vi "TESTE.vi"() -> ()   [LabVIEW 2018]
uses:
  CCDCamera/CCDCamera.lvclass
  <userlib>/atmcd32d.llb/Shutter_mode typedef.ctl
  <userlib>/atmcd32d.llb/HSSpeed_type typedef.ctl
  <userlib>/atmcd32d.llb/AcquisitionMode_mode typedef.ctl
  <userlib>/atmcd32d.llb/TriggerMode_mode typedef.ctl
  <userlib>/atmcd32d.llb/ReadMode_mode typedef.ctl
  <userlib>/atmcd32d.llb/Shutter_type typedef.ctl
  <userlib>/gfitsio/gfitsio.lvlib
  <userlib>/gfitsio/cfitsio-bitpix.ctl
  <userlib>/gfitsio/gfitsio-write-key-string.vi
  <userlib>/gfitsio/gfitsio-write-image-subset-variant.vi
  Save Image/Save Image.lvclass
  Sync Box/Sync Box.lvclass
panel:
  out "data out":string
  in  "Array 2":u16[](array[numeric])
  in  "CCD Config":T1={"Exposure Time"=0.1, "Pre-amp gain"=0, "Readout Rate"=0, "EM Mode"=0, "EM Gain"=2, "Binning"=1, "Initial Line"=1, "Initial Cloumn"=1, "Final Line"=1024, "Final Column"=1024, "Kinetic Series Length"=1, "Shutter Mode"=0, "Cooler ON/OFF"=0, "Temperature"=20, "Image Name"="", "Image Path"="", "Current Temperature"=0, "Temperatue Status"="", "Serial Number"=0, "#image"=1} {"Pre-amp gain" items=["Gain 1", "Gain 2"]; "Readout Rate" items=["1 MHz", "10 MHz", "20 MHz", "30 MHz"]; "EM Mode" items=["Electron Multiplying", "Conventional"]}
  in  "Array":u16[][][](array[numeric])=[[[1, 2], [3, 4]], [[5, 6], [7, 8]], [[4, 7], [8, 7]]]
  out "array":u16[][][](array[numeric])
  out "last":u8
  out "first":u8
  in  "CCDCamera.lvclass":refnum<class "CCDCamera.lvclass">
  out "speed":sgl format="%.2f"
  in  "Header Contents":T2={"FILENAME"=["FILENAME", "Image", "File name at acquisition"], "OBSERVER"=["OBSERVER", "Anonymous", "Name of the observer"], "PROGRID"=["PROGRID", "2018A-001", "Program ID"], "OBJECT"=["OBJECT", "UNDEFINED", "Object name"], "NIGHTDIR"=["NIGHTDIR", "C:\\Users\\observer\\Desktop\\SPARC4 Acquisition Control\\Imagens\\", "Night directory name "], "CHANNEL"=["CHANNEL", "1", "Instrument channel"], "INSTRUME"=["INSTRUME", "SPARC4", "Instrument"], "NEXPSEQ"=["NEXPSEQ", "1", "Total number of exposures in sequence"], "SEQINDEX"=["SEQINDEX", "1", "Exposure index in the sequence"], "OBSTYPE"=["OBSTYPE", "BIAS", "Image type: OBJECT, BIAS, FLAT, ARC, DARK"], "READMOD"=["READMOD", "Normal", "Read out mode: fast, normal, slow"], "READMODE"=["READMODE", "Image", "CCD read mode"], "ACQMODE"=["ACQMODE", "Kinetic", "Acquisition Mode"], "PREAMP"=["PREAMP", "Gain 1", "Pre-amplifier gain"], "READOUT"=["READOUT", "30 MHz", "Readout Rate"], "VSHIFT"=["VSHIFT", "4.33", "Vertical Shift Speed"], "TRIGGER"=["TRIGGER", "Internal", "Trigger Mode"], "EMMODE"=["EMMODE", "Electron Multiplying", "Output amplifier mode"], "EMGAIN"=["EMGAIN", "2", "EM Gain"], "VBIN"=["VBIN", "1", "Vertical binning"], "HBIN"=["HBIN", "1", "Horizontal binning"], "INITLINE"=["INITLIN", "1", "Initial Line"], "INITCOL"=["INITCOL", "1", "Initial Column"], "FINALLIN"=["FINALIN", "1024", "Final Line"], "FINALCOL"=["FINALCOL", "1", "Final Column"], "KSERLEN"=["KSERLEN", "CLOSED", "Kinetic Series Length"], "SHUTTER"=["SHUTTER", "50", "Shutter Mode (OPEN, CLOSED, or AUTO) "], "OPENSHT"=["OPENSHT", "50", "Time to open the shutter (ms) "], "CLOSESHT"=["CLOSESHT", "2019-03-14T14:55:35.63", "Time to close the shutter (ms)"], "DATE"=["DATE", "3.38", "Date of the acquired image (YY/MM/DD:HH:MM:SS.sss"], "GAIN"=["GAIN", "0.05", "Gain (e-/ADU)"], "GAINERR "=["GAINERR", "6.55", " Gain error (e-/ADU)"], "RDNOISE"=["RDNOISE", "0.02", "Read noise (e-)"], "RNOISERR"=["RNOISERR", "OFF", "Read noise error (e-)"], "SKYFIBER"=["SKYFIBER", "OFF", "Sky fiber: ON or OFF"], "CALFIBER"=["CALFIBER", "2017-10-01T20", "Calibration Fiber: ON or OFF"], "UTDATE"=["UTDATE", "2017-10-01T17", "UT date at start of exposure"], "LOCTIME"=["LOCTIME", "58027.500000", "LT date at start of exposure"], "MJD"=["MJD", "-45.57972", "Modified Julian Date at start of exposure"], "OBSLON"=["OBSLON", "-22.53444", "Observatory East Longitude"], "OBSLAT"=["OBSLAT", "1864.0", "Observatory Latitude"], "OBSALT"=["OBSALT", "0", "Observatory elevation above sea level (m)"], "EXPTIME"=["EXPTIME", "0000:00.000", "Exposure time (s)"], "TELRA"=["TELRA", "+00:00:00.000", "TCS right ascension: HH:MM:SS.SSS"], "TELDEC"=["TELDEC", "00:00:00.000", "TCS declination: +-DD:MM:SS.SSS"], "RA"=["RA", "+00:00:00.000", "Requested right Ascension: HH:MM:SS.SSS"], "DEC"=["DEC", "128.84946", "Requested Declination: +- DD:MM:SS.SSS"], "RA_DEG"=["RA_DEG", "+19.648717", "Requested Right Ascension (deg)"], "DEC_DEG"=["DEC_DEG", "2000.00", "Requested Declination (deg)"], "EPOCH"=["EPOCH", "+01:13:05.98", "Epoch for Target coordinates"], "HA"=["HA", "1.2183292", "Hour Angle (Sexagesimal)"], "HAD"=["HAD", "1.085", "Hour Angle (deg)"], "AIRMASS"=["AIRMASS", "1.060", "Mean airmass for the observation"], "AMSTART"=["AMSTART", "1.114", "Airmass at start of exposure"], "AMEND"=["AMEND", "0.000000", "Airmass at end of exposure"], "XOFFSET"=["XOFFSET", "0.000000", "Telescope RA offset in arcsec"], "YOFFSET"=["YOFFSET", "14.6415392418", "Telescope DEC offset in arcsec"], "PA"=["PA", "-3.53", "Current Rotator Position Angle (degree)"], "CAMFOC"=["CAMFOC", "-3.53", "Camera focus position (mm)"], "TELFOC"=["TELFOC", "23:17:24.8", "Telescope focus position (mm)"], "TCSUT"=["TCSUT", "23:12:32.5", "TCS Universal Time"], "TCSST"=["TCSST", "15.0", "TCS Sideral Time"], "MOONDIST"=["MOONDIST", "60.0", "Moon angular distance to object (deg)"], "MOONALT"=["MOONALT", "15.0", "Moon elevation above horizon (deg)"], "MOONPHAS"=["MOONPHAS", "30.0", "Moon phase (deg)"], "ADC"=["ADC", "OFF", "Atmospheric Dispersion Corrector: ON or OFF"], "ADCSPEED"=["ADCSPEED", "0", "ADC motor speed (rpm)"], "CALMIRR"=["CALMIRR", "OUT", "Calibration mirror position: IN or OUT"], "GUIDING"=["GUIDING", "OFF", "Guider status: ON or OFF"], "GUIDTEXP"=["GUIDTEXP", "0", "Guider exposure time (s)"], "GUIDFREQ"=["GUIDFREQ", "0", "Guiding frequency (Hz)"], "GUIDOBJX"=["GUIDOBJX", "102.5", "Guiding object x position (pixel)"], "GUIDOBJY"=["GUIDOBJY", "300.3", "Guiding object y position (pixel)"], "AVGYCORR"=["AVGYCORR", "2.3", "Average correction in RA (arcsec)"], "AVGXCORR"=["AVGXCORR", "1.3", "Average correction in DEC (arcsec)"], "GFOCUS"=["GFOCUS", "3.0", "Guider focus position (mm)"], "THARLAMP"=["THARLAMP", "OFF", "Thorium-Argon lamp state: ON or OFF"], "HALLAMP"=["HALLAMP", "OFF", "Halogen lamp state: ON or OFF"], "AGITATOR"=["AGITATOR", "OFF", "Fiber agitator: ON or OFF"], "THARMIRR"=["THARMIRR", "OFF", "Th-Ar mirror position: SPECTROGRAPH or TELESCOPE"], "DSTATUS"=["DSTATUS", "SPECTROGRAPH", "Dome Status: OPEN or CLOSED"], "DTEMP"=["DTEMP", "OPEN", "Dome temperature (deg C)"], "DHUM"=["DHUM", "0.00000", "Dome humidity (per cent)"], "DLAMP"=["DLAMP", "10.0", "Dome lamp: ON or OFF"], "DFLAT"=["DFLAT", "82.0", "Dome flat lamp: ON or OFF"], "TEMPEXT"=["TEMPEXT", "OFF", "External temperature (deg C)"], "PRESSURE"=["PRESSURE", "OFF", "Pressure (mbar)"], "HUMIDITY"=["HUMIDITY", "10.0", "Humidity (per cent)"], "WINDDIR"=["WINDDIR", "742.00", "Wind direction: North-eastward (deg)"], "WSPEED"=["WSPEED", "92.00", "Wind Speed (km/h)"], "DPOS"=["DPOS", "30.2", "Dome position (deg)"], "SHTTTL"=["SHTTTL", "TTL LOW", "Shutter TTL"]}
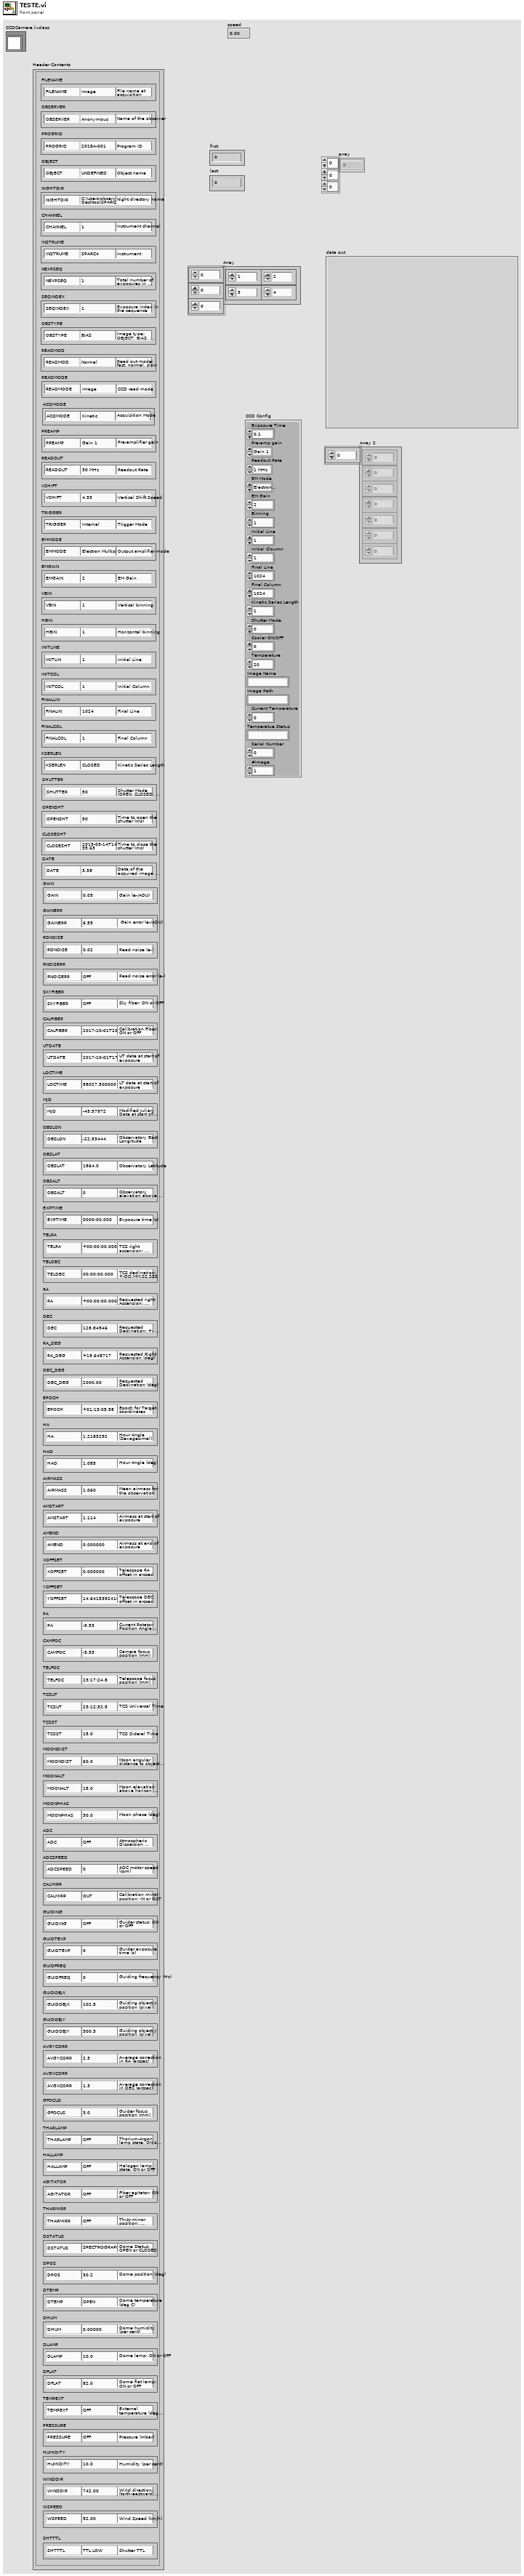
[diagram p1: front panel]
types:
  T1 = cluster{"Exposure Time":sgl, "Pre-amp gain":u8, "Readout Rate":u8, "EM Mode":u8, "EM Gain":u16, "Binning":u16, "Initial Line":u16, "Initial Cloumn":u16, "Final Line":u16, "Final Column":u16, "Kinetic Series Length":u32, "Shutter Mode":u8, "Cooler ON/OFF":u8, "Temperature":i8, "Image Name":string, "Image Path":string, "Current Temperature":i16, "Temperatue Status":string, "Serial Number":u16, "#image":u32}
  T2 = cluster{"FILENAME":string[], "OBSERVER":string[], "PROGRID":string[], "OBJECT":string[], "NIGHTDIR":string[], "CHANNEL":string[], "INSTRUME":string[], "NEXPSEQ":string[], "SEQINDEX":string[], "OBSTYPE":string[], "READMOD":string[], "READMODE":string[], "ACQMODE":string[], "PREAMP":string[], "READOUT":string[], "VSHIFT":string[], "TRIGGER":string[], "EMMODE":string[], "EMGAIN":string[], "VBIN":string[], "HBIN":string[], "INITLINE":string[], "INITCOL":string[], "FINALLIN":string[], "FINALCOL":string[], "KSERLEN":string[], "SHUTTER":string[], "OPENSHT":string[], "CLOSESHT":string[], "DATE":string[], "GAIN":string[], "GAINERR ":string[], "RDNOISE":string[], "RNOISERR":string[], "SKYFIBER":string[], "CALFIBER":string[], "UTDATE":string[], "LOCTIME":string[], "MJD":string[], "OBSLON":string[], "OBSLAT":string[], "OBSALT":string[], "EXPTIME":string[], "TELRA":string[], "TELDEC":string[], "RA":string[], "DEC":string[], "RA_DEG":string[], "DEC_DEG":string[], "EPOCH":string[], "HA":string[], "HAD":string[], "AIRMASS":string[], "AMSTART":string[], "AMEND":string[], "XOFFSET":string[], "YOFFSET":string[], "PA":string[], "CAMFOC":string[], "TELFOC":string[], "TCSUT":string[], "TCSST":string[], "MOONDIST":string[], "MOONALT":string[], "MOONPHAS":string[], "ADC":string[], "ADCSPEED":string[], "CALMIRR":string[], "GUIDING":string[], "GUIDTEXP":string[], "GUIDFREQ":string[], "GUIDOBJX":string[], "GUIDOBJY":string[], "AVGYCORR":string[], "AVGXCORR":string[], "GFOCUS":string[], "THARLAMP":string[], "HALLAMP":string[], "AGITATOR":string[], "THARMIRR":string[], "DSTATUS":string[], "DTEMP":string[], "DHUM":string[], "DLAMP":string[], "DFLAT":string[], "TEMPEXT":string[], "PRESSURE":string[], "HUMIDITY":string[], "WINDDIR":string[], "WSPEED":string[], "DPOS":string[], "SHTTTL":string[]}
  T3 = typedef "Shutter_mode typedef.ctl" = enum16{"Auto", "Open", "Close", "N/A (3)", "Open FVB Series", "Open Any Series"}
  T4 = typedef "AcquisitionMode_mode typedef.ctl" = enum16{"Reserved (0)", "Single Scan", "Accumulate", "Kinetics", "Fast Kinetics", "Run Till Abort", "Reserved (6)", "Reserved (7)", "Reserved (8)", "Time Delayed Integration"}
  T5 = typedef "TriggerMode_mode typedef.ctl" = enum16{"Internal", "External", "N/A (2)", "N/A (3)", "N/A (4)", "N/A (5)", "External Start", "External Exposure (Bulb)", "N/A (8)", "External FVB EM", "Software", "N/A (11)", "External Charge Shifting"}
  T6 = typedef "ReadMode_mode typedef.ctl" = enum16{"Full Vertical Binning", "Multi-Track", "Random-Track", "Single-Track", "Image"}
  T7 = typedef "Shutter_type typedef.ctl" = enum16{"TTL Low", "TTL High"}
  T8 = typedef "HSSpeed_type typedef.ctl" = enum16{"EM Amp", "Conventional Amp"}
  T9 = enum16{"open", "open or create", "create", "create or replace"}
  T10 = enum16{"open", "open or create", "create or replace", "create", "open (read only)"}
  T11 = typedef "gfitsio.lvlib/cfitsio-bitpix.ctl" = i32
  T12 = typedef "gfitsio.lvlib/gfitsio-refnum.ctl" = refnum<k1>
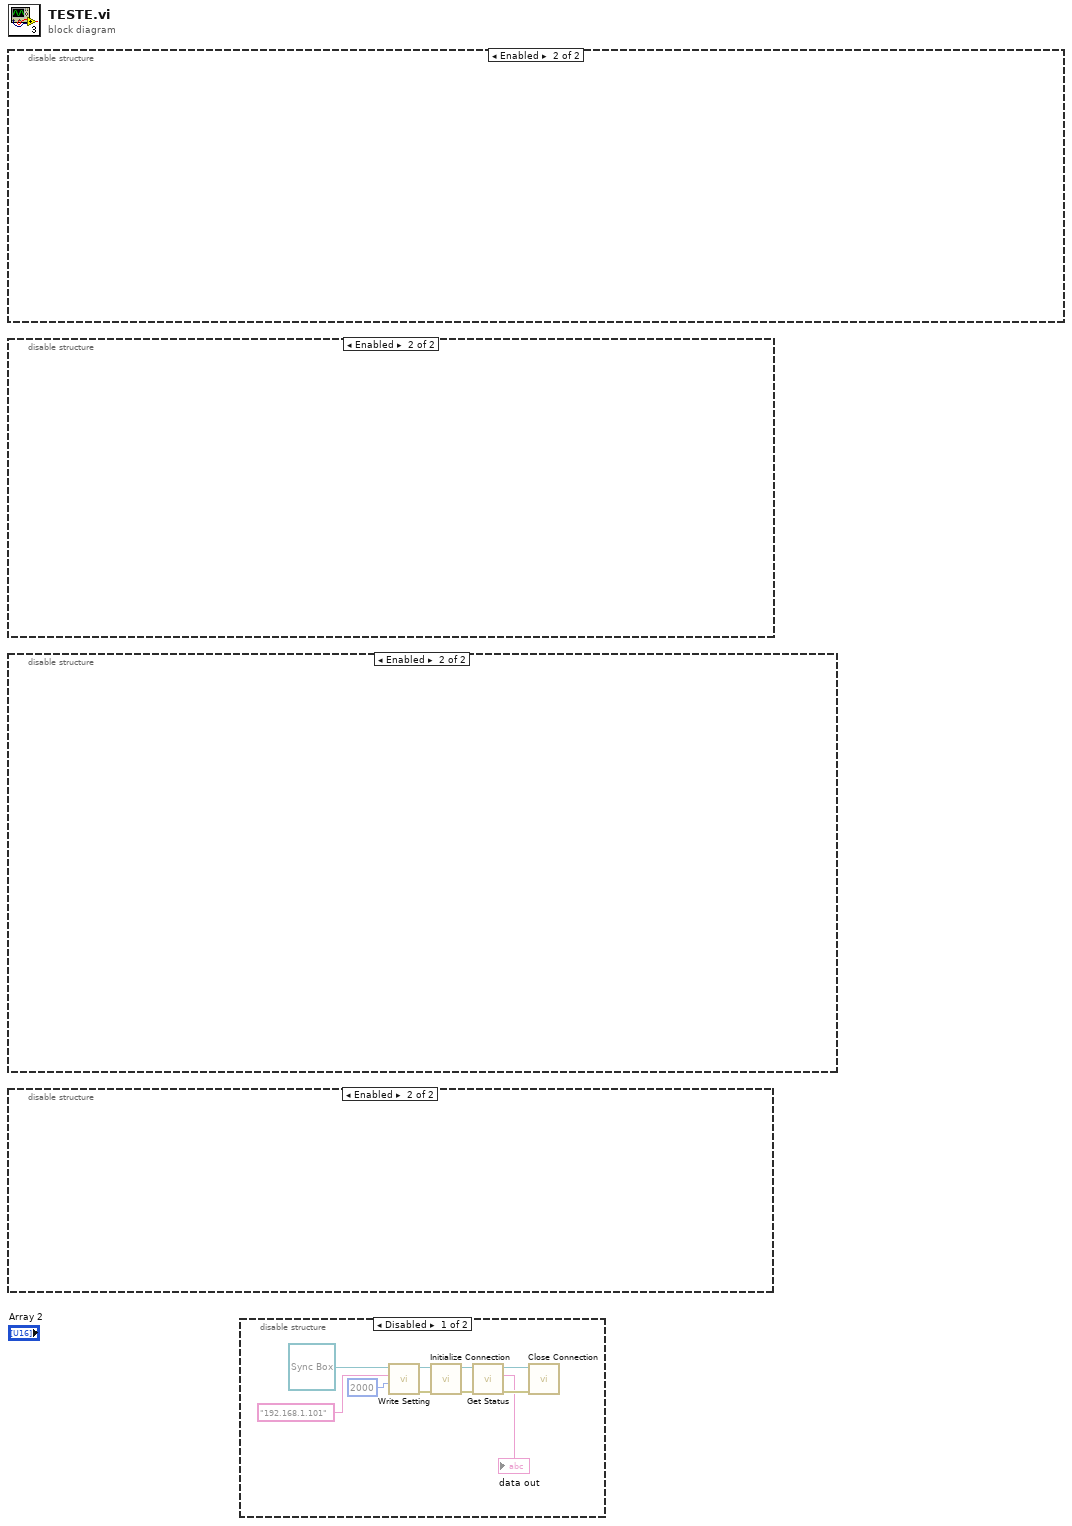
[diagram p0: block diagram]
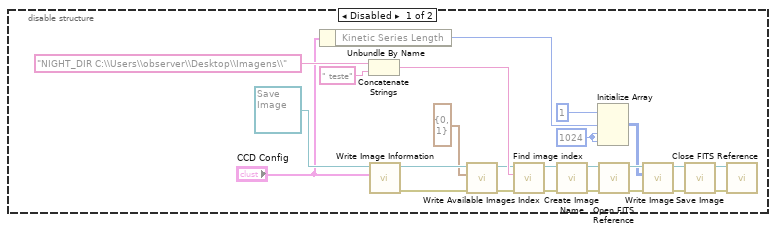
[diagram p3: hidden frame]
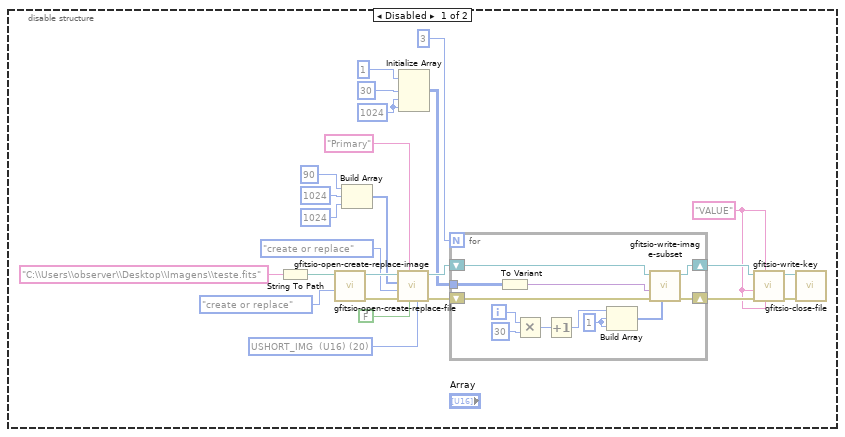
[diagram p4: hidden frame]
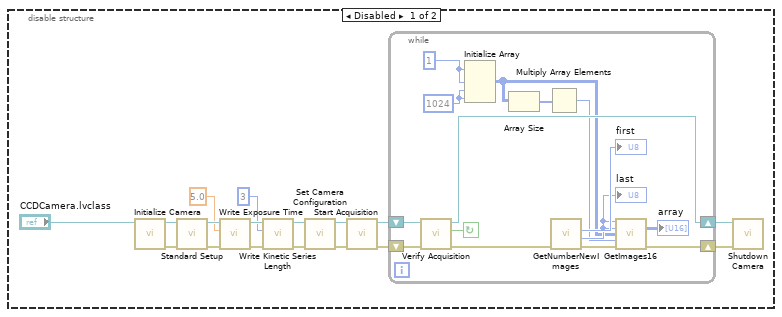
[diagram p5: hidden frame]
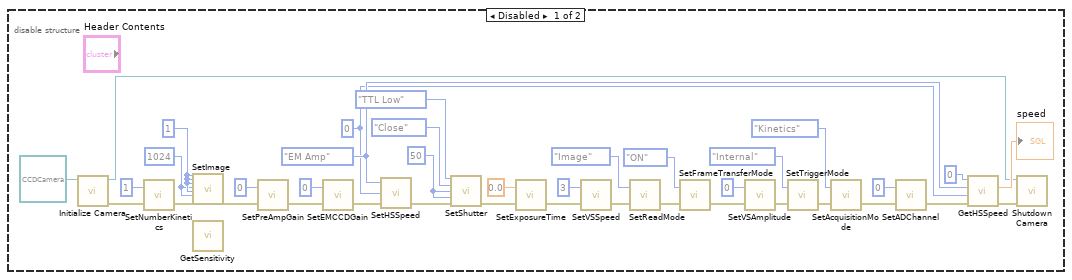
[diagram p6: hidden frame]
diagram:
  n1 = disable-structure shown="Enabled" {
    frame Disabled {
      w2 = HSSpeed_type_typedef."EM Amp" ("type")
      w1 = 0 ("index")
      w12 = 1024 ("number")
      w13 = 1 ("number")
      w28 = 50 ("openingtime")
      n2 = call "Initialize Camera.vi"("CCDCamera in"=refnum<class "CCDCamera.lvclass"> refnum ("CCDCamera.lvclass")) -> ("error out"=w5:errorcluster, "CCDCamera out"=w3:refnum<class "CCDCamera.lvclass">)  [unwired: 9 in]
      n3 = call <userlib>:"SetNumberKinetics.vi"("error in (no error)"=w5, "number"=1) -> ("error out"=w31:errorcluster)  [unwired: 1 out]
      n4 = call <userlib>:"SetImage.vi"("hbin"=w13, "vbin"=w13, "hstart"=w13, "hend"=w12, "vstart"=w13, "vend"=w12, "error in (no error)"=w31) -> ("error out"=w30:errorcluster)  [unwired: 19 in, 1 out]
      n5 = call <userlib>:"GetSensitivity.vi"() -> ()  [unwired: 5 in, 3 out]
      n6 = call <userlib>:"SetPreAmpGain.vi"("error in (no error)"=w30, "index"=0) -> ("error out"=w32:errorcluster)  [unwired: 1 out]
      n7 = call <userlib>:"SetEMCCDGain.vi"("error in (no error)"=w32, "gain"=0) -> ("error out"=w33:errorcluster)  [unwired: 1 out]
      n8 = call <userlib>:"SetHSSpeed.vi"("error in (no error)"=w33, "index"=w1, "type"=w2) -> ("error out"=w34:errorcluster)  [unwired: 1 in, 1 out]
      n9 = call <userlib>:"SetShutter.vi"("type"=Shutter_type_typedef."TTL Low", "mode"=Shutter_mode_typedef."Close", "closingtime"=w28, "openingtime"=w28, "error in (no error)"=w34) -> ("error out"=w17:errorcluster)  [unwired: 9 in, 1 out]
      n10 = call <userlib>:"SetExposureTime.vi"("error in (no error)"=w17, "time"=sgl 0.0) -> ("error out"=w16:errorcluster)  [unwired: 1 out]
      n11 = call <userlib>:"SetVSSpeed.vi"("error in (no error)"=w16, "index"=3) -> ("error out"=w35:errorcluster)  [unwired: 1 out]
      n12 = call <userlib>:"SetReadMode.vi"("error in (no error)"=w35, "mode"=ReadMode_mode_typedef."Image") -> ("error out"=w25:errorcluster)  [unwired: 1 out]
      n13 = call <userlib>:"SetFrameTransferMode.vi"("error in (no error)"=w25, "mode"=enum16{"OFF", "ON"}."ON") -> ("error out"=w23:errorcluster)  [unwired: 1 out]
      n14 = call <userlib>:"SetVSAmplitude.vi"("error in (no error)"=w23, "amplitude"=0) -> ("error out"=w21:errorcluster)  [unwired: 1 out]
      n15 = call <userlib>:"SetTriggerMode.vi"("error in (no error)"=w21, "mode"=TriggerMode_mode_typedef."Internal") -> ("error out"=w20:errorcluster)  [unwired: 1 out]
      n16 = call <userlib>:"SetAcquisitionMode.vi"("error in (no error)"=w20, "mode"=AcquisitionMode_mode_typedef."Kinetics") -> ("error out"=w15:errorcluster)  [unwired: 1 out]
      n17 = call <userlib>:"SetADChannel.vi"("error in (no error)"=w15, "channel"=0) -> ("error out"=w7:errorcluster)  [unwired: 1 out]
      n18 = call <userlib>:"GetHSSpeed.vi"("error in (no error)"=w7, "index"=w1, "type"=w2, "channel"=0) -> ("error out"=w4:errorcluster, "speed"=→"speed":sgl)  [unwired: 1 in, 1 out]
      n19 = call "Shutdown Camera.vi"("error in (no error)"=w4, "CCDCamera in"=w3) -> ()  [unwired: 8 in, 2 out]
    }
    frame Enabled {
    }
  }
  n20 = disable-structure shown="Enabled" {
    frame Disabled {
      n21 = call "Initialize Camera.vi"("CCDCamera in"="CCDCamera.lvclass") -> ("error out"=w45:errorcluster, "CCDCamera out"=w54:refnum<class "CCDCamera.lvclass">)  [unwired: 9 in]
      n22 = call "Standard Setup.vi"("error in (no error)"=w45, "CCDCamera in"=w54) -> ("error out"=w46:errorcluster, "CCDCamera out"=w53:refnum<class "CCDCamera.lvclass">)  [unwired: 8 in]
      n23 = call "Write Exposure Time.vi"("error in (no error)"=w46, "Exposure Time"=5.0, "CCDCamera in"=w53) -> ("error out"=w40:errorcluster, "CCDCamera out"=w43:refnum<class "CCDCamera.lvclass">)  [unwired: 7 in]
      n24 = call "Write Kinetic Series Length.vi"("error in (no error)"=w40, "Kinetic Series Length"=3, "CCDCamera in"=w43) -> ("error out"=w41:errorcluster, "CCDCamera out"=w42:refnum<class "CCDCamera.lvclass">)  [unwired: 7 in]
      n25 = call "Set Camera Configuration.vi"("error in (no error)"=w41, "CCDCamera in"=w42) -> ("error out"=w47:errorcluster, "CCDCamera out"=w52:refnum<class "CCDCamera.lvclass">)  [unwired: 8 in]
      n26 = call "Start Acquisition.vi"("error in (no error)"=w47, "CCDCamera in"=w52) -> ("error out"=w48:errorcluster, "CCDCamera out"=w51:refnum<class "CCDCamera.lvclass">)  [unwired: 8 in]
      n27 = while {
        shift-right: [w69] -> w50
        shift-left: w51 -> [w70]
        shift-right: [w63] -> w49
        shift-left: w48 -> [w68]
        stop <- w67 continue-if-true
        w61 = 1024
        w60 = 1
        n28 = call "Verify Acquisition.vi"("error in (no error)"=w68, "CCDCamera in"=w70) -> ("error out"=w66:errorcluster, "Acquiring"=w67:bool, "CCDCamera out"=w69:refnum<class "CCDCamera.lvclass">)  [unwired: 7 in]
        n29 = Initialize Array(w60, w60, w61, w61) -> (w59:i32[][][])
        n30 = Array Size(array=w59) -> (size(s)=w58:i32[])
        n31 = Multiply Array Elements(1:w58) -> (0:w57:i32)
        n32 = call <userlib>:"GetNumberNewImages.vi"("error in (no error)"=w66) -> ("error out"=w64:errorcluster, "last"=w62:i32, "first"=→"first":u32)  [unwired: 3 in, 1 out]
        "last" <- w62
        n33 = call <userlib>:"GetImages16.vi"("first"=w62, "last"=w62, "array"=w59, "size"=w57, "error in (no error)"=w64) -> ("array"=→"array":u16[][][], "error out"=w63:errorcluster)  [unwired: 6 in, 3 out]
      }
      n34 = call "Shutdown Camera.vi"("error in (no error)"=w49, "CCDCamera in"=w50) -> ()  [unwired: 8 in, 2 out]
    }
    frame Enabled {
    }
  }
  n35 = disable-structure shown="Enabled" {
    frame Disabled {
      w71 = 1024
      w76 = "VALUE" ("keyname")
      w88 = T11 20 items=["<invalid type>"=0, "BYTE_IMG  (U8)"=8, "SHORT_IMG  (I16)"=16, "USHORT_IMG  (U16)"=20, "LONG_IMG  (I32)"=32, "ULONG_IMG  (U32)"=40, "FLOAT_IMG  (SGL)"=-32, "DOUBLE_IMG  (DBL)"=-64] ("image data type")
      n36 = String To Path(string="C:\\Users\\observer\\Desktop\\Imagens\\teste.fits" ("prompt")) -> (path=w93:path)
      n37 = call <userlib>:"gfitsio-open-create-replace-file.vi"("function (open)"=T10."create or replace", "file path (dialog if empty)"=w93) -> ("error out"=w95:errorcluster, "gfits refnum"=w94:T12)  [unwired: 7 in, 1 out]
      n38 = Build Array(90, 1024, 1024) -> (w85:i32[])
      n39 = call <userlib>:"gfitsio-open-create-replace-image.vi"("image data type"=w88, "advisory dialog? (display:T)"=FALSE, "hdu name (dialog if empty)"="Primary" ("prompt"), "error in (no error)"=w95, "function (create or replace)"=T9."create or replace" ("function (open or create)"), "naxes"=w85, "gfits refnum"=w94) -> ("error out"=w86:errorcluster, "dup gfits refnum"=w87:T12)  [unwired: 2 in, 1 out]
      n40 = Initialize Array(1, 30, w71, w71) -> (w73:i32[][][])
      n41 = for {
        N: 3 -> [_]
        shift-right: [w106] -> w77
        shift-left: w87 -> [w105]
        shift-right: [w107] -> w78
        shift-left: w86 -> [w104]
        tunnel: w73 -> [w99]
        i -> [w98]
        w101 = 1
        n42 = To Variant(anything=w99) -> (Variant=w103:variant)
        n43 = Multiply(x=w98, y=30) -> (x*y=w96:i32)
        n44 = Increment(x=w96) -> (x+1=w102:i32)
        n45 = Build Array(w102, w101, w101) -> (w100:i32[])
        n46 = call-poly <userlib>:"gfitsio-write-image-subset.vi"("fpixel"=w100, "error in (no error)"=w104, "data"=w103, "gfits refnum"=w105) -> ("error out"=w107:errorcluster, "dup gfits refnum"=w106:T12)  [unwired: 6 in]
      }
      n47 = call-poly <userlib>:"gfitsio-write-key.vi"("comment"=w76, "keyname"=w76, "error in (no error)"=w78, "value"=w76, "gfits refnum"=w77) -> ("error out"=w79:errorcluster, "dup gfits refnum"=w80:T12)  [unwired: 5 in]
      n48 = call <userlib>:"gfitsio-close-file.vi"("error in (no error)"=w79, "gfits refnum"=w80) -> ()  [unwired: 8 in, 2 out]
    }
    frame Enabled {
    }
  }
  n49 = disable-structure shown="Enabled" {
    frame Disabled {
      w122 = 1024
      n50 = Unbundle By Name("CCD Config") -> ("Kinetic Series Length"=w108:u32)
      n51 = Concatenate Strings("NIGHT_DIR C:\\Users\\observer\\Desktop\\Imagens\\", " teste") -> (w115:string)
      n52 = call "Write Image Information.vi"("CCD Config"="CCD Config", "Save Image in"=refnum<class "Save Image.lvclass"> refnum ("Save Image.lvclass")) -> ("error out"=w111:errorcluster, "Save Image out"=w114:refnum<class "Save Image.lvclass">)  [unwired: 8 in]
      n53 = call "Write Available Images Index.vi"("error in (no error)"=w111, "available images index"=cluster{"previous":u16, "next":u16} {"previous"=0, "next"=1}, "Save Image in"=w114) -> ("error out"=w112:errorcluster, "Save Image out"=w113:refnum<class "Save Image.lvclass">)  [unwired: 7 in]
      n54 = call "Find image index.vi"("error in (no error)"=w112, "Message"=w115, "Save Image in"=w113) -> ("error out"=w118:errorcluster, "Save Image in"=w119:refnum<class "Save Image.lvclass">)  [unwired: 7 in]
      n55 = call "Create Image Name.vi"("error in (no error)"=w118, "Save Image in"=w119) -> ("error out"=w130:errorcluster, "Save Image out"=w131:refnum<class "Save Image.lvclass">)  [unwired: 8 in]
      n56 = Initialize Array(u16 1, w108, w122, w122) -> (w120:u16[][][])
      n57 = call "Open FITS Reference.vi"("error in (no error)"=w130, "Save Image in"=w131) -> ("error out"=w127:errorcluster, "Save Image out"=w128:refnum<class "Save Image.lvclass">)  [unwired: 8 in]
      n58 = call "Write Image.vi"("error in (no error)"=w127, "Image"=w120, "Save Image in"=w128) -> ("error out"=w125:errorcluster, "Save Image out"=w126:refnum<class "Save Image.lvclass">)  [unwired: 7 in]
      n59 = call "Save Image.vi"("error in (no error)"=w125, "Save Image in"=w126) -> ("error out"=w123:errorcluster, "Save Image out"=w124:refnum<class "Save Image.lvclass">)  [unwired: 8 in]
      n60 = call "Close FITS Reference.vi"("error in (no error)"=w123, "Save Image in"=w124) -> ()  [unwired: 8 in, 2 out]
    }
    frame Enabled {
    }
  }
  n61 = disable-structure shown="Disabled" {
    frame Disabled {
      n62 = call "Write Setting.vi"("Remote Port"=u32 2000, "Address"="192.168.1.101", "Sync Box in"=refnum<class "Sync Box.lvclass"> refnum ("Sync Box.lvclass")) -> ("error out"=w136:errorcluster, "Sync Box out"=w141:refnum<class "Sync Box.lvclass">)  [unwired: 7 in]
      n63 = call "Initialize Connection.vi"("error in (no error)"=w136, "Sync Box in"=w141) -> ("error out"=w138:errorcluster, "Sync Box out"=w140:refnum<class "Sync Box.lvclass">)  [unwired: 7 in, 1 out]
      n64 = call "Get Status.vi"("error in (no error)"=w138, "Sync Box in"=w140) -> ("error out"=w137:errorcluster, "data out"=→"data out":string, "Sync Box out"=w139:refnum<class "Sync Box.lvclass">)  [unwired: 7 in]
      n65 = call "Close Connection.vi"("error in (no error)"=w137, "Sync Box in"=w139) -> ()  [unwired: 8 in, 2 out]
    }
    frame Enabled {
    }
  }
